vi "QT_MovieGetFrame.vi"(0 "QT Ref In":T2, 1 "Frame Access":T1, 2 "Frame ID":i32, 5 "error in":errorcluster, 8 "Private":T3) -> (14 "QT Ref Out":T2, 16 "Image Out":T4 {"Dialogs" format="%.0b"}, 19 "error out":errorcluster)   [LabVIEW 2024]
uses:
  <userlib>/ImageProcessing/QTLIB_2595_LV86/QT_Selector.ctl
  <userlib>/ImageProcessing/QTLIB_2595_LV86/QT_Image.ctl
  <userlib>/ImageProcessing/QTLIB_2595_LV86/QT_FrameSelector.ctl
  <userlib>/ImageProcessing/QTLIB_2595_LV86/QT_Private.ctl
  <userlib>/ImageProcessing/QTLIB_2595_LV86/QT_Ref.ctl
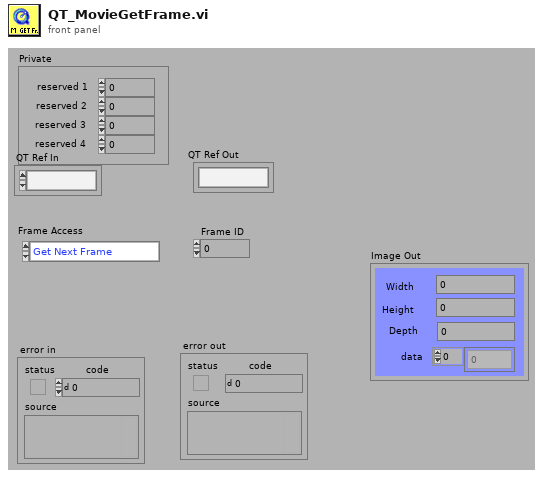
[diagram p1: front panel]
types:
  T1 = typedef "QT_FrameSelector.ctl" = enum32{"Get Next Frame", "Get Prev Frame", "Get Last Frame", "Get First Frame", "Get Frame ID", "Get Frame at Time", "reserved"}
  T2 = typedef "QT_Ref.ctl" = refnum<k1>
  T3 = typedef "QT_Private.ctl" = cluster{"reserved 1":i32, "reserved 2":i32, "reserved 3":i32, "reserved 4":i32}
  T4 = typedef "QT_Image.ctl" = cluster{"Width":i32, "Height":i32, "Depth":i32, "data":u8[], "Compressed data":u8[], "Color table":u32[], "Duration":i32, "Options":i32, "Timestamp":i32, "ID":i32, "Reserved":i32, "Dialogs":u32}
  T5 = typedef "QT_Selector.ctl" = enum32{"do nothing", "Get all Sources", "Get Source info", "Open Image", "Save Image to File", "Effect", "Close", "SG Grab", "Compress in Memory", "Decompress to Memory", "New Movie", "Open Movie", "Add Frame", "Get Frame", "Close Movie", "Get QT & CIN info", "SG init", "SG Close", "Open sound file", "Close sound file", "Read sound data", "Write sound data", "Import sound", "Export sound", "Add sound to movie", "Get sound from movie", "reserved", "reserved 1", "reserved 2"}
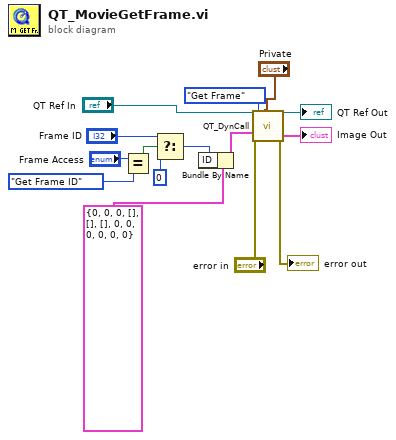
[diagram p0: block diagram]
diagram:
  n1 = Equal?(x="Frame Access", y=QT_FrameSelector."Get Frame ID" ("Frame Access")) -> (x = y?=w3:bool)
  n2 = Select(t="Frame ID", s=w3, f=0) -> (s? t:f=w6:i32)
  n3 = Bundle By Name(cluster=T4 {"Width"=0, "Height"=0, "Depth"=0, "data"=[], "Compressed data"=[], "Color table"=[], "Duration"=0, "Options"=0, "Timestamp"=0, "ID"=0, "Reserved"=0, "Dialogs"=0} ("Image in"), "ID"=w6) -> (w7:T4)
  n4 = call <userlib>:"QT_DynCall.vi"("QT Ref In"="QT Ref In", "Image in"=w7, "error in (no error)"="error in", "Selector"=QT_Selector."Get Frame", "Private"="Private") -> ("QT Ref Out"=→"QT Ref Out":T2, "Image/Movie Out"=→"Image Out":T4, "error out"=→"error out":errorcluster)  [unwired: 7 in, 13 out]
